vi "Create Stop Event.vi"(8 "error in (no error)":errorcluster, 11 "EventHandler":refnum<class "IEventHandler.lvclass">) -> (0 "error out":errorcluster, 3 "EventHandler":refnum<class "IEventHandler.lvclass">)   [LabVIEW 2015, in "ActorEvents.lvlib" / "IEventHandler.lvclass"]
uses:
  IEventHandler.lvclass
  IEventHandler.lvclass/IEventHandler.ctl
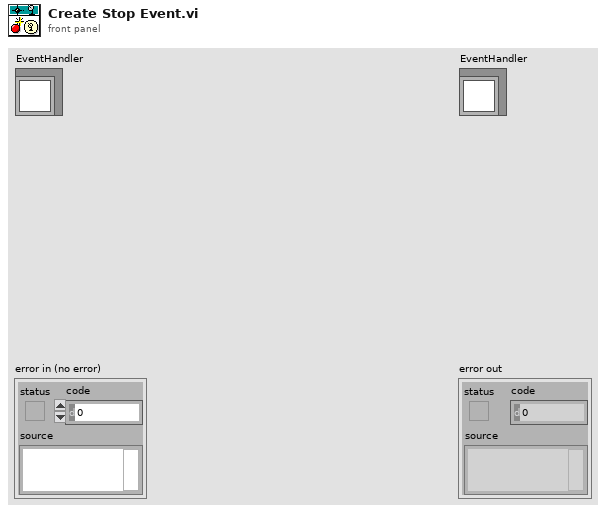
[diagram p1: front panel]
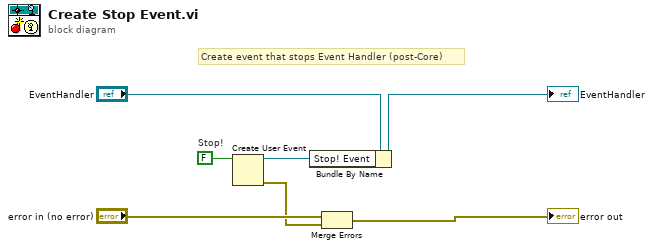
[diagram p0: block diagram]
diagram:
  w4 = FALSE  # Stop!
  # "Create event that stops Event Handler (post-Core)"
  n1 = Create User Event(user event datatype=w4) -> (user event=w3:refnum<user-event>, error out=w1:errorcluster)  [unwired: 1 in]
  n2 = Bundle By Name(cluster="EventHandler", "Stop! Event"=w3) -> (→"EventHandler":refnum<class "IEventHandler.lvclass">)
  n3 = Merge Errors("error in (no error)", w1) -> (→"error out":errorcluster)
